vi "写入系列号对话框.vi"() -> ()   [LabVIEW 2016, in "斯坦道总磷总氮.lvlib"]
panel:
  in  "布尔":bool
  out "序列号":string
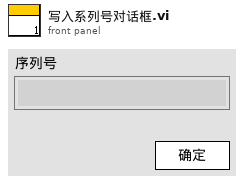
[diagram p1: front panel]
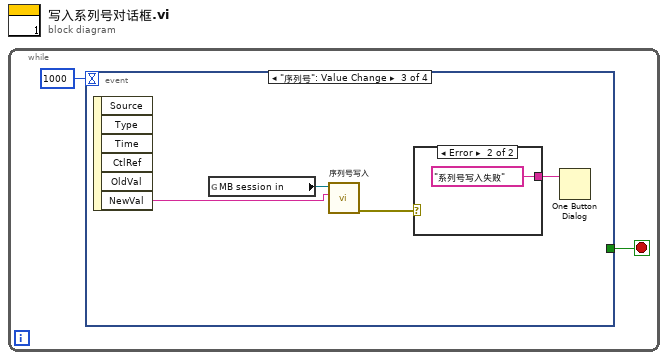
[diagram p0: block diagram]
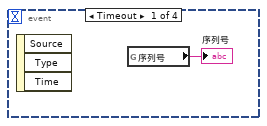
[diagram p2: hidden frame]
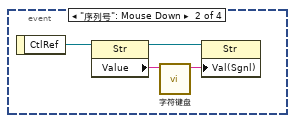
[diagram p3: hidden frame]
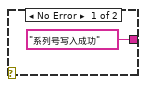
[diagram p4: hidden frame]
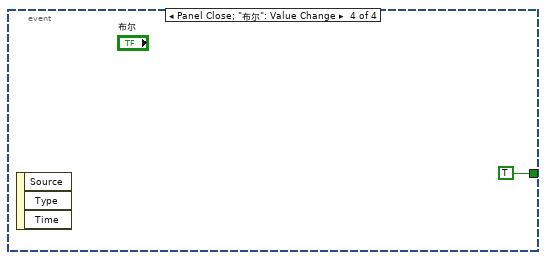
[diagram p5: hidden frame]
diagram:
  n1 = while {
    stop <- w2 stop-if-true
    n2 = event shown="[2] \"序列号\": Value Change" {
      selector: _ -> [_ _ _ _]
      dyn-events: _ -> [_ _ _ _]
      timeout: 1000 -> [_ _ _ _]
      tunnel: [_ _ _ TRUE] -> w2
      event Timeout {
        n3 = event-data() -> ()  [unwired: 1 in, 3 out]
        n4 = global read "VAR总磷总氮全局变量.vi" "序列号"() -> (→"序列号":string)
      }
      event "序列号": Mouse Down {
        n5 = event-data() -> ("CtlRef"=w7:refnum<vi>)  [unwired: 1 in]
        n6 = property class="Str"(reference=w7) -> (reference out=w4:refnum<vi>, "Value"=w6:string)  [unwired: 1 in, 1 out]
        n7 = call "字符键盘.vi"("Old String"=w6) -> ("String"=w5:string)  [unwired: 10 in]
        n8 = property class="Str"(reference=w4, "Val(Sgnl)"=w5) -> ()  [unwired: 1 in, 2 out]
      }
      event "序列号": Value Change {
        n9 = event-data() -> ("NewVal"=w11:string)  [unwired: 1 in, 5 out]
        n10 = global read "VAR总磷总氮全局变量.vi" "MB session in"() -> (w10:refnum<class "MB_Master.lvclass">)
        n11 = call "序列号写入.vi"("序列号"=w11, "MB session in"=w10) -> ("error out"=w9:errorcluster)  [unwired: 8 in, 1 out]
        n12 = case shown="Error" w9 {
          tunnel: ["系列号写入成功" "系列号写入失败"] -> w8
          frame No Error {
          }
          frame Error {
          }
        }
        n13 = One Button Dialog(message=w8) -> ()  [unwired: 1 in, 1 out]
      }
      event Panel Close; "布尔": Value Change {
        n14 = event-data() -> ()  [unwired: 1 in, 3 out]
      }
    }
  }
